vi "lab 1.3.vi"() -> ()   [LabVIEW 2020]
uses:
  <vilib>/Analysis/2dsp.llb/1D Convolution (DBL).vi
  <vilib>/measure/maspectr.llb/FFT Spectrum (Mag-Phase) for 1 Chan.vi
  <vilib>/express/express analysis/Spectral/Block/exnSpectralBlock spectral measurements peak poly.vi
  <vilib>/express/express analysis/Spectral/Block/exnSpectralBlock spectral measurements peak WFM.vi
  <vilib>/express/express analysis/Spectral/XNode/ExpressSpectralMeasurementsBlockNode.xnode
  <vilib>/measure/NI_MABase.lvlib
  <vilib>/Analysis/NI_AALPro.lvlib
  <vilib>/measure/NI_MAPro.lvlib
panel:
  out "Waveform Graph 6":dbl[](graph)
  out "Waveform Graph 5":dbl[](graph)
  out "Waveform Graph 4":dbl[](graph)
  out "Waveform Graph 3":cluster{"f0":dbl, "df":dbl, "magnitude":dbl[]}(graph)
  out "Waveform Graph 2":waveform(dbl)(graph)
  out "Waveform Graph":cluster{"f0":dbl, "df":dbl, "magnitude":dbl[]}(graph)
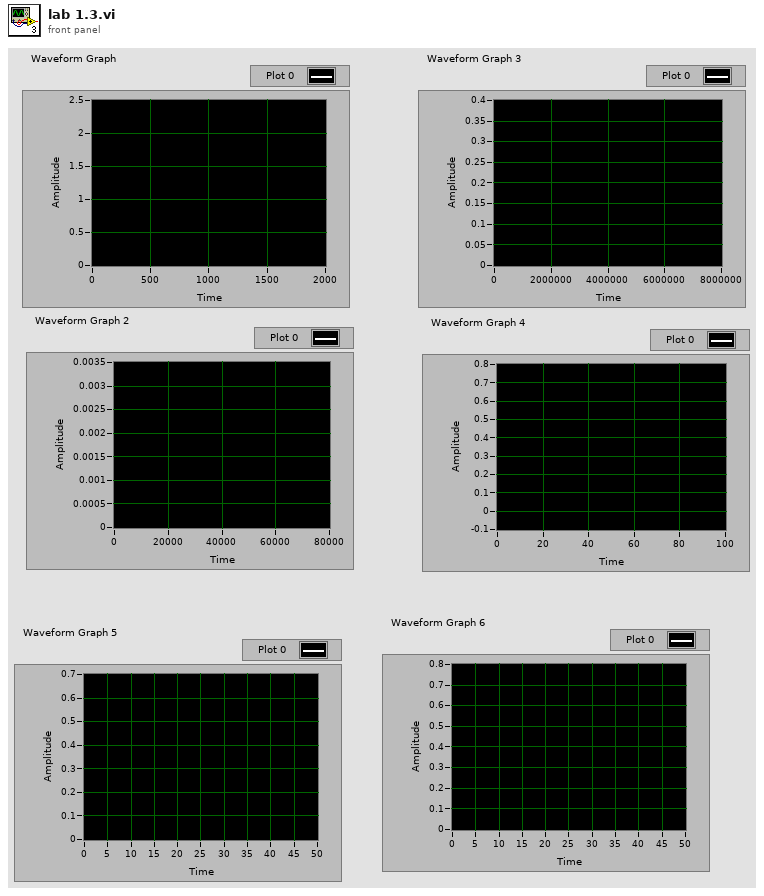
[diagram p1: front panel]
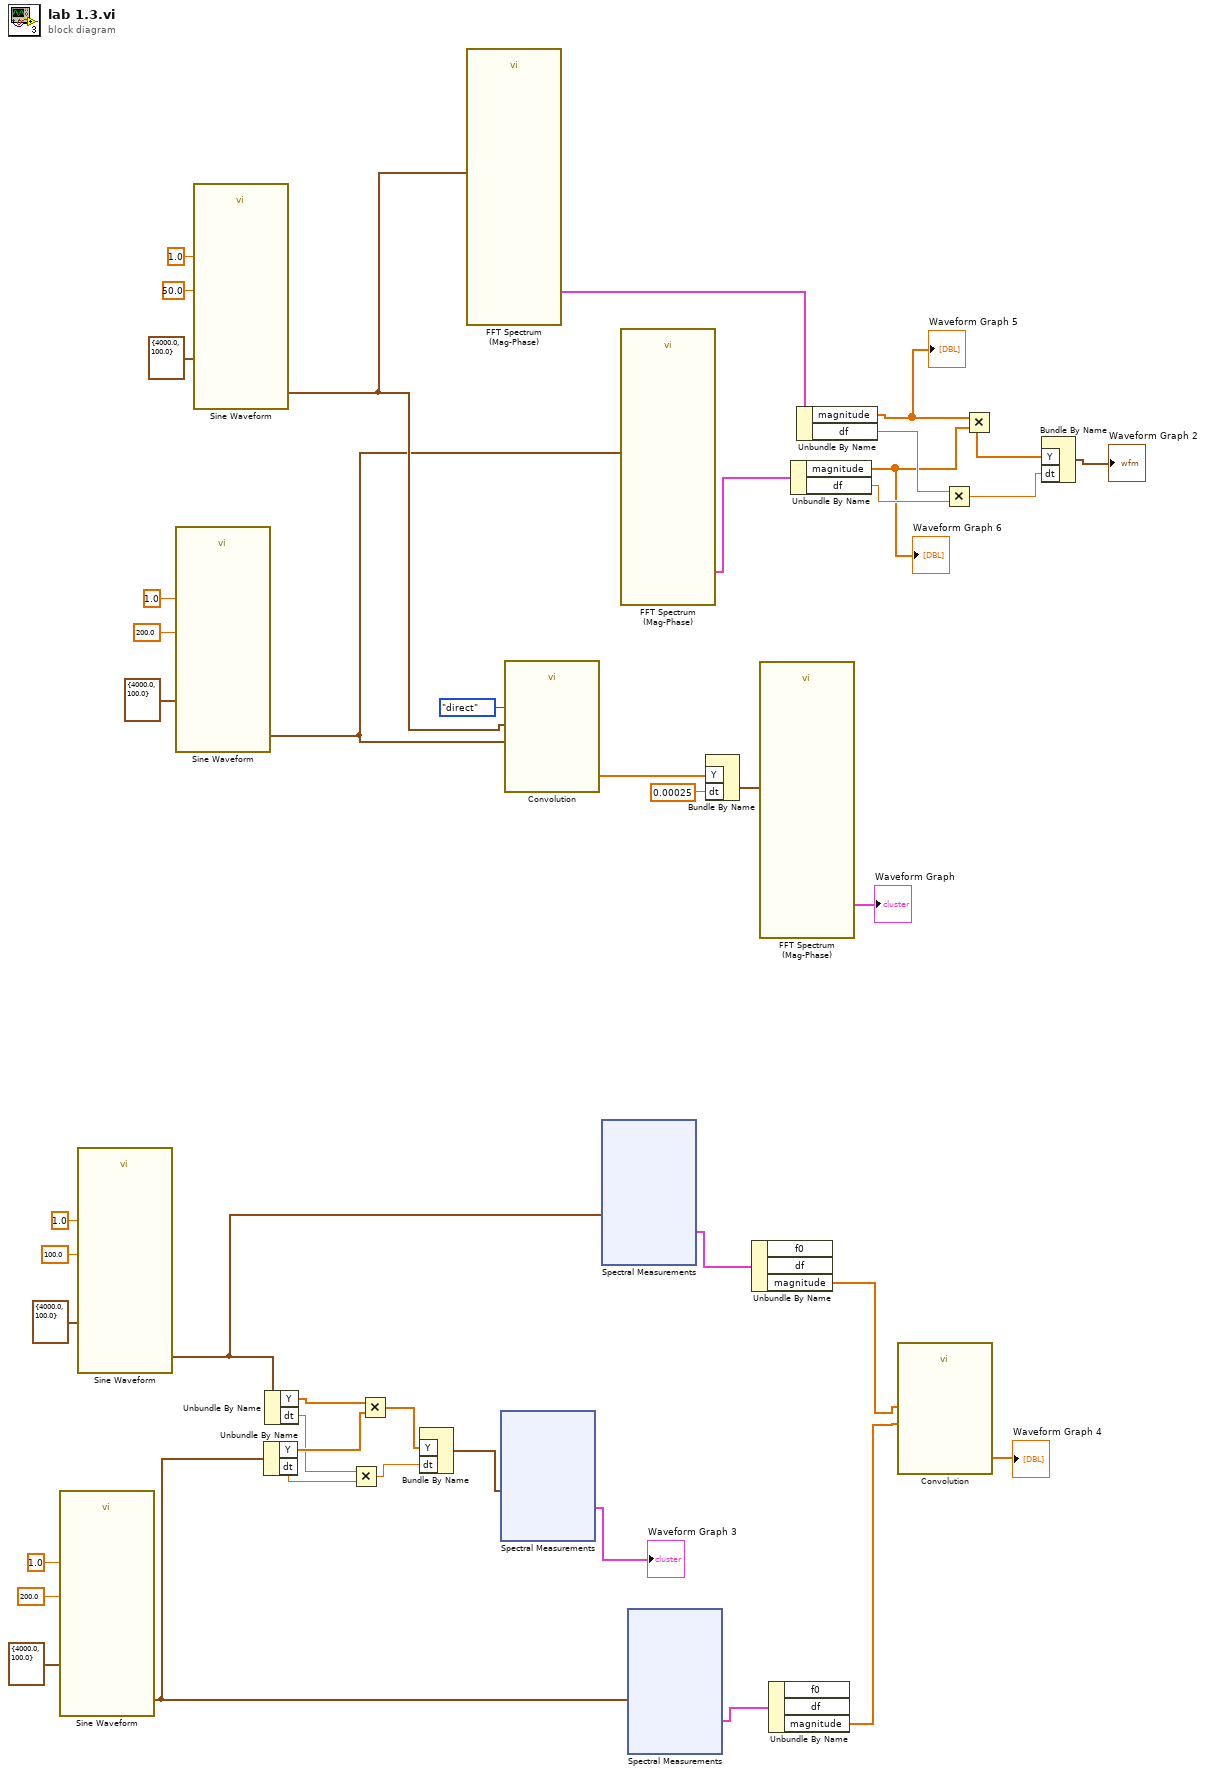
[diagram p0: block diagram]
diagram:
  n1 = call <vilib>:"Sine Waveform.vi"("sampling info"=cluster{"Fs":dbl, "#s":dbl} {"Fs"=4000.0, "#s"=100.0}, "amplitude"=1.0, "frequency"=200.0) -> ("signal out"=w8:waveform(dbl))  [unwired: 7 in, 1 out]
  n2 = call <vilib>:"Sine Waveform.vi"("sampling info"=cluster{"Fs":dbl, "#s":dbl} {"Fs"=4000.0, "#s"=100.0}, "amplitude"=1.0, "frequency"=100.0) -> ("signal out"=w9:waveform(dbl))  [unwired: 7 in, 1 out]
  n3 = call <vilib>:"Sine Waveform.vi"("sampling info"=cluster{"Fs":dbl, "#s":dbl} {"Fs"=4000.0, "#s"=100.0}, "amplitude"=1.0, "frequency"=200.0) -> ("signal out"=w31:waveform(dbl))  [unwired: 7 in, 1 out]
  n4 = call <vilib>:"Sine Waveform.vi"("sampling info"=cluster{"Fs":dbl, "#s":dbl} {"Fs"=4000.0, "#s"=100.0}, "amplitude"=1.0, "frequency"=50.0) -> ("signal out"=w32:waveform(dbl))  [unwired: 7 in, 1 out]
  n5 = Unbundle By Name(w8) -> ("Y"=w19:dbl[], "dt"=w14:dbl)
  n6 = Unbundle By Name(w9) -> ("Y"=w20:dbl[], "dt"=w15:dbl)
  n7 = Multiply(x=w15, y=w14) -> (x*y=w13:dbl)
  n8 = Multiply(x=w20, y=w19) -> (x*y=w18:dbl[])
  n9 = Bundle By Name("Y"=w18, "dt"=w13) -> (w17:waveform(dbl))  [unwired: 1 in]
  n10 = call-poly <vilib>:"FFT Spectrum (Mag-Phase).vi"("time signal"=w32) -> ("magnitude"=w30:cluster{"f0":dbl, "df":dbl, "magnitude":dbl[]})  [unwired: 6 in, 4 out]
  n11 = xnode "Spectral Measurements"("Signals"=w17) -> ("FFT - (Peak)"=→"Waveform Graph 3":cluster{"f0":dbl, "df":dbl, "magnitude":dbl[]})  [unwired: 1 in, 2 out]
  n12 = call-poly <vilib>:"Convolution.vi"("algorithm"=enum32{"direct", "frequency domain"}."direct", "Y"=w31, "X"=w32) -> ("X * Y"=w36:dbl[])  [unwired: 7 in, 1 out]
  n13 = xnode "Spectral Measurements"("Signals"=w9) -> ("FFT - (Peak)"=w7:cluster{"f0":dbl, "df":dbl, "magnitude":dbl[]})  [unwired: 1 in, 2 out]
  n14 = call-poly <vilib>:"FFT Spectrum (Mag-Phase).vi"("time signal"=w31) -> ("magnitude"=w29:cluster{"f0":dbl, "df":dbl, "magnitude":dbl[]})  [unwired: 6 in, 4 out]
  n15 = xnode "Spectral Measurements"("Signals"=w8) -> ("FFT - (Peak)"=w6:cluster{"f0":dbl, "df":dbl, "magnitude":dbl[]})  [unwired: 1 in, 2 out]
  n16 = Bundle By Name("Y"=w36, "dt"=0.00025) -> (w34:waveform(dbl))  [unwired: 1 in]
  n17 = Unbundle By Name(w7) -> ("magnitude"=w4:dbl[])  [unwired: 2 out]
  n18 = call-poly <vilib>:"FFT Spectrum (Mag-Phase).vi"("time signal"=w34) -> ("magnitude"=→"Waveform Graph":cluster{"f0":dbl, "df":dbl, "magnitude":dbl[]})  [unwired: 6 in, 4 out]
  n19 = Unbundle By Name(w6) -> ("magnitude"=w5:dbl[])  [unwired: 2 out]
  n20 = Unbundle By Name(w29) -> ("magnitude"=w1:dbl[], "df"=w11:dbl)
  "Waveform Graph 6" <- w1
  n21 = Unbundle By Name(w30) -> ("magnitude"=w2:dbl[], "df"=w12:dbl)
  "Waveform Graph 5" <- w2
  n22 = call-poly <vilib>:"Convolution.vi"("Y"=w5, "X"=w4) -> ("X * Y"=→"Waveform Graph 4":dbl[])  [unwired: 8 in, 1 out]
  n23 = Multiply(x=w12, y=w11) -> (x*y=w10:dbl)
  n24 = Multiply(x=w2, y=w1) -> (x*y=w28:dbl[])
  n25 = Bundle By Name("Y"=w28, "dt"=w10) -> (→"Waveform Graph 2":waveform(dbl))  [unwired: 1 in]
